vi "MeasureTempArduino 2.vi"() -> ()   [LabVIEW 2015]
uses:
  <vilib>/ni845x/ni845x.llb/ni845xControl.ctl
  <vilib>/addons/control/pid/pid.llb/PID Control Input Filter (DBL).vi
  <vilib>/addons/control/pid/autopid.llb/PID Online Autotuning (Relay Feedback).vi
  <vilib>/addons/control/pid/pid.llb/PID Advanced (DBL).vi
  <vilib>/addons/control/pid/NI_PID_pid.lvlib
  <vilib>/addons/control/pid/NI_PID_autopid.lvlib
  <vilib>/MakerHub/LINX/LMH-LINX.lvlib
panel:
  in  "Channel":i32
  in  "Arduino Port":refnum<visa-resource-name>="N/A"
  in  "Address 2":u8=80 format="%.0x"
  in  "device reference":T1
  in  "Output range":cluster{"output high":dbl, "output low":dbl}={"output high"=5.0, "output low"=0.0} {"output low" format="%.2f"; "output high" format="%.2f"}
  in  "Autotuning Parameters":T2={"type of controller"=enum."PID", "relay cycles"=3, "relay amplitude"=1.0, "control specifications"=enum."Normal", "PV noise level"=0.1} {"PV noise level" format="%.2f"; "relay amplitude" format="%.2f"}
  out "MV":dbl(graph)
  in  "Autotune":bool=TRUE
  out "tuning completed?":bool
  out "tuned PID gains":T3
  in  "Accept gain":bool=TRUE
  in  "SP":dbl=50.0 format="%#_13g"
  out "SP and PV":cluster{"data":dbl, "SP":dbl}(graph)
  in  "MV(sec)":dbl format="%#_13g"
  in  "PID gains":T4={"Proportional gain Kc"=0.180743, "Integral time Ti (sec)"=0.463767, "Derivative time Ti (sec)"=0.111304}
  in  "Stop":bool
  out "PV":dbl format="%0.2f"
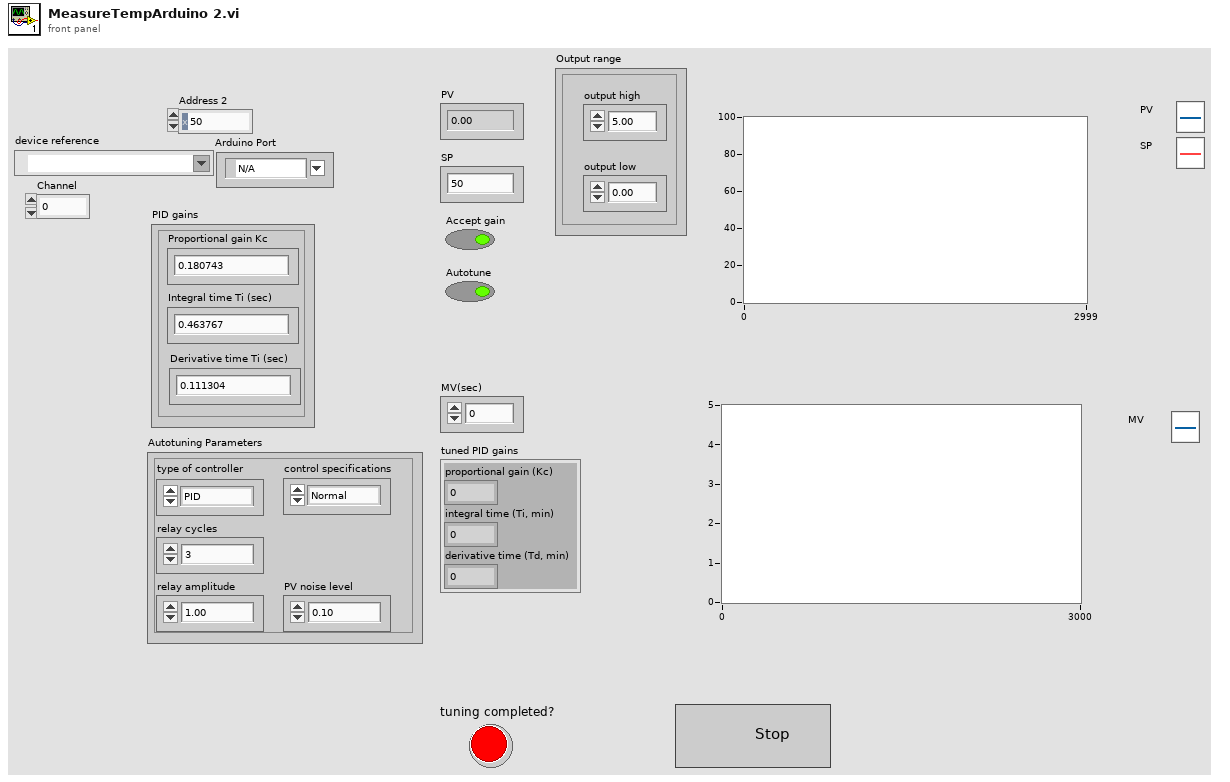
[diagram p1: front panel]
types:
  T1 = typedef "ni845xControl.ctl" = refnum<k21>
  T2 = cluster{"type of controller":enum16{"P", "PI", "PID"}, "relay cycles":i32, "relay amplitude":dbl, "control specifications":enum16{"Fast", "Normal", "Slow"}, "PV noise level":dbl}
  T3 = cluster{"proportional gain (Kc)":dbl, "integral time (Ti, min)":dbl, "derivative time (Td, min)":dbl}
  T4 = cluster{"Proportional gain Kc":dbl, "Integral time Ti (sec)":dbl, "Derivative time Ti (sec)":dbl}
  T5 = typedef "LMH-LINX.lvlib/LINX Ref.ctl" = cluster{"Platform":T6, "Interface":T7, "LINX Device Config":T8}
  T6 = typedef "LMH-LINX.lvlib/Platform.ctl" = enum16{"LINX", "myRIO"}
  T7 = typedef "LMH-LINX.lvlib/Interface.ctl" = enum16{"Serial", "TCP"}
  T8 = typedef "LMH-LINX.lvlib/Device.lvlib/LINX Device Config.ctl" = cluster{"Interface":T7, "COM Port":refnum<visa-resource-name>, "TCP Configuration":T9, "Device Family":u8, "Device ID":u8, "Device Name":string, "TCP Ref":refnum<k5>, "Channels":T10}
  T9 = typedef "LMH-LINX.lvlib/Device.lvlib/TCP Config.ctl" = cluster{"IP Address":string, "Port":u16}
  T10 = typedef "LMH-LINX.lvlib/Channels.ctl" = cluster{"DI":u8[], "DO":u8[], "AI":u8[], "AO":u8[], "PWM":u8[], "QE":u8[], "UART":u8[], "I2C 2":u8[], "SPI":u8[], "CAN":u8[], "Servo":u8[], "AI Ref (V)":dbl, "AO Ref (V)":dbl, "AO Resolution (Bits)":u8}
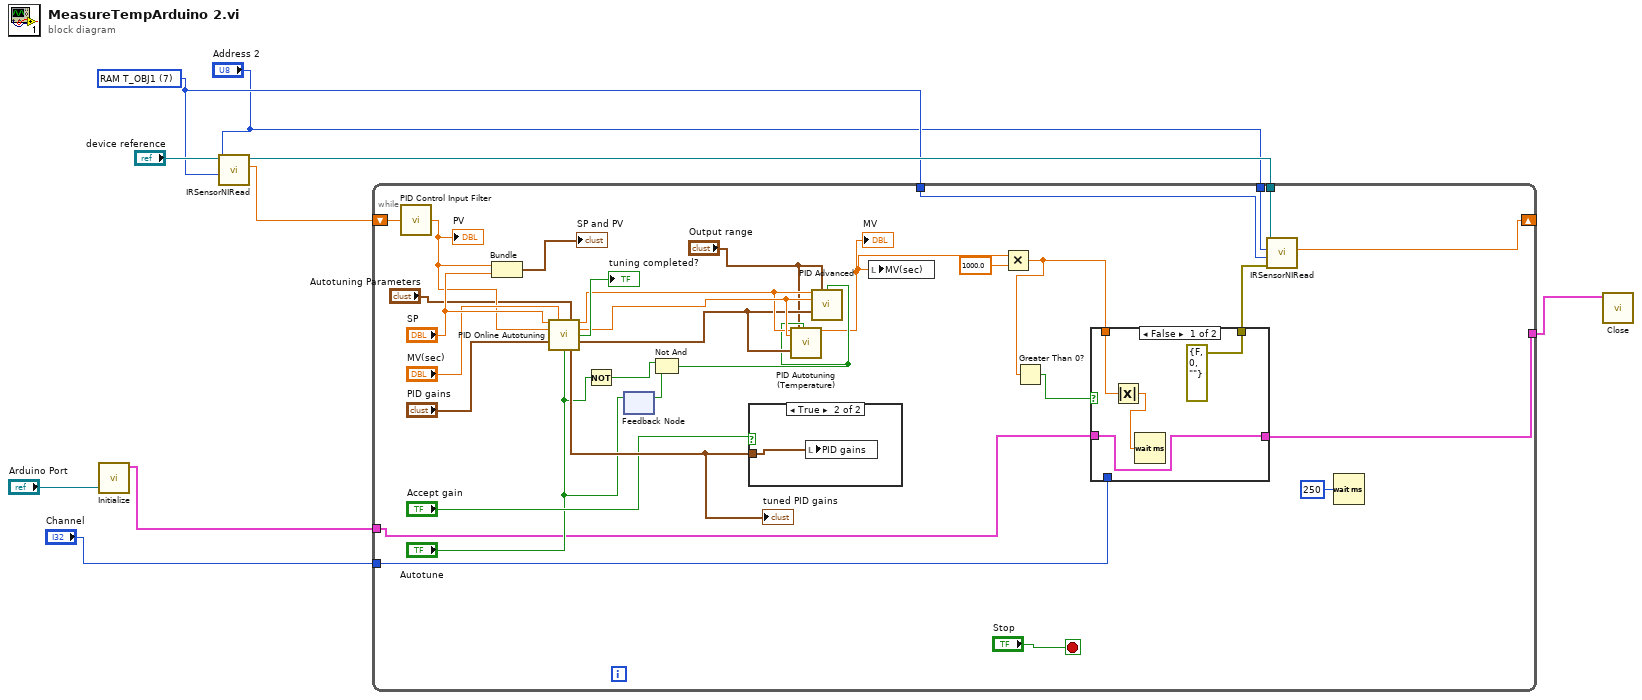
[diagram p0: block diagram]
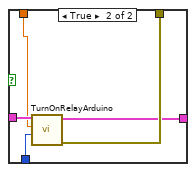
[diagram p2: hidden frame]
diagram:
  w7 = u8 7 items=["RAM IR raw  Ch1"=4, "RAM IR raw  Ch2"=5, "RAM T_A"=6, "RAM T_OBJ1"=7, "RAM T_OBJ2"=8, "EEPROM_To_max"=32, "EEPROM_To_min"=33, "EEPROM_PWM_CTRL"=34, "EEPROM_Ta_range"=35, "EEPROM_Emissivity_CorrCoeff"=36, "EEPROM_SMBus Address"=46, "EEPROM_ConfigReg"=37] ("Melexis_Cmmds")
  n1 = call <vilib>:"Initialize.vi"("Serial Port"="Arduino Port") -> ("LINX Ref"=w4:T5)  [unwired: 8 in, 2 out]
  n2 = call "IRSensorNIRead.vi"("Melexis_Cmmds"=w7, "Address"="Address 2", "device reference"="device reference") -> ("Temperature"=w2:dbl, "device reference out"=w8:T1)  [unwired: 6 in, 1 out]
  n3 = while {
    shift-right: [w11] -> _
    shift-left: w2 -> [w30]
    tunnel: w8 -> [w26]
    tunnel: "Address 2" -> [w25]
    tunnel: w7 -> [w24]
    tunnel: w4 -> [w13]
    tunnel: "Channel" -> [w12]
    tunnel: [w10] -> w1
    stop <- "Stop" stop-if-true
    n4 = call-poly <vilib>:"PID Control Input Filter.vi"("input"=w30) -> ("output"=w29:dbl)  [unwired: 4 in]
    "PV" <- w29
    n5 = Bundle("output"=w29, "SP"="SP") -> (→"SP and PV":cluster{"output":dbl, "SP":dbl})  [unwired: 1 in]
    n6 = call-poly <vilib>:"PID Online Autotuning.vi"("setpoint"="SP", "manipulated variable"="MV(sec)", "autotuning parameters"="Autotuning Parameters", "process variable"=w29, "PID gains in"="PID gains", "autotune? (F)"="Autotune") -> ("setpoint out"=w20:dbl, "process variable out"=w21:dbl, "tuning completed?"=→"tuning completed?":bool, "PID gains out"=w19:T3, "tuned PID gains"=w40:T3)  [unwired: 5 in]
    "tuned PID gains" <- w40
    n7 = Not(x="Autotune") -> (.not. x?=w32:bool)
    n8 = feedback #1() -> (w31:bool)  [unwired: 1 in]
    n9 = feedback-in #1("Autotune") -> ()
    n10 = Not And(1:w31, 2:w32) -> (0:w18:bool)
    n11 = case shown="True" "Accept gain" {
      tunnel: w40 -> [_ w51]
      frame False {
      }
      frame True {
        n12 = local write "PID gains"(w51) -> ()
      }
    }
    n13 = call <vilib>:"PID Autotuning (Temperature).vi"("desired temperature"=w20, "measured temperature"=w21, "PID gains in"=w19, "output range"="Output range", "auto? (T)"=w18) -> ("output"=w16:dbl)  [unwired: 11 in, 3 out]
    "MV" <- w16
    n14 = call-poly <vilib>:"PID Advanced.vi"("setpoint"=w20, "output range"="Output range", "auto? (T)"=w18, "process variable"=w21, "PID gains"=w19) -> ()  [unwired: 9 in, 2 out]
    n15 = local write "MV(sec)"(w16) -> ()
    n16 = Multiply(x=w16, y=1000.0) -> (x*y=w15:dbl)
    n17 = Greater Than 0?(x=w15) -> (x > 0?=w14:bool)
    n18 = case shown="False" w14 {
      tunnel: [errorcluster {"status"=FALSE, "code"=0, "source"=""} ("error out") w47] -> w27
      tunnel: w15 -> [w44 w49]
      tunnel: w13 -> [w42 w50]
      tunnel: w12 -> [_ w48]
      tunnel: [w42 w46] -> w10
      frame False {
        n19 = Absolute Value(x=w44) -> (abs(x)=w43:dbl)
        n20 = Wait (ms)(milliseconds to wait=w43) -> ()  [unwired: 1 out]
      }
      frame True {
        n21 = call "TurnOnRelayArduino.vi"("channel"=w48, "duration"=w49, "LINX Resource"=w50) -> ("error out"=w47:errorcluster, "LINX Resource Out"=w46:T5)  [unwired: 7 in]
      }
    }
    n22 = call "IRSensorNIRead.vi"("error in (no error)"=w27, "Melexis_Cmmds"=w24, "Address"=w25, "device reference"=w26) -> ("Temperature"=w11:dbl)  [unwired: 5 in, 2 out]
    n23 = Wait (ms)(milliseconds to wait=u32 250) -> ()  [unwired: 1 out]
  }
  n24 = call <vilib>:"Close.vi"("LINX Resource"=w1) -> ()  [unwired: 9 in, 2 out]
